vi "nanos.get.vi"(8 "error in (no error)":errorcluster, 11 "endingTimestamp in":refnum<class "endingTimestamp.lvclass">) -> (0 "error out":errorcluster, 2 "nanos":i64, 3 "endingTimestamp out":refnum<class "endingTimestamp.lvclass">)   [LabVIEW 2020, in "nominal types.lvlib" / "timestampManifest.lvlib" / "endingTimestamp.lvclass"]
uses:
  endingTimestamp.lvclass
  endingTimestamp.lvclass/endingTimestamp.ctl
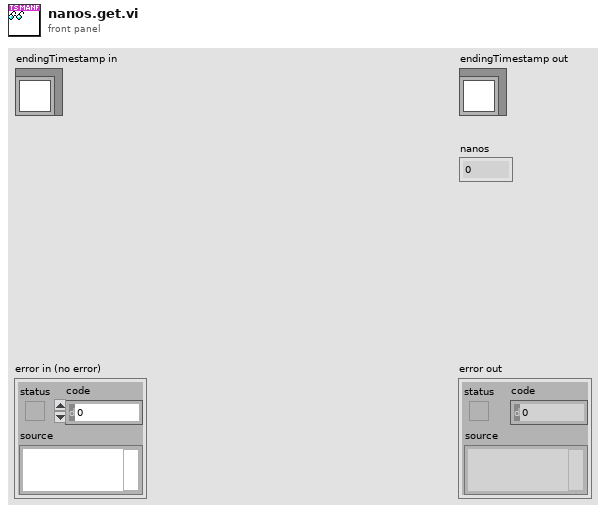
[diagram p1: front panel]
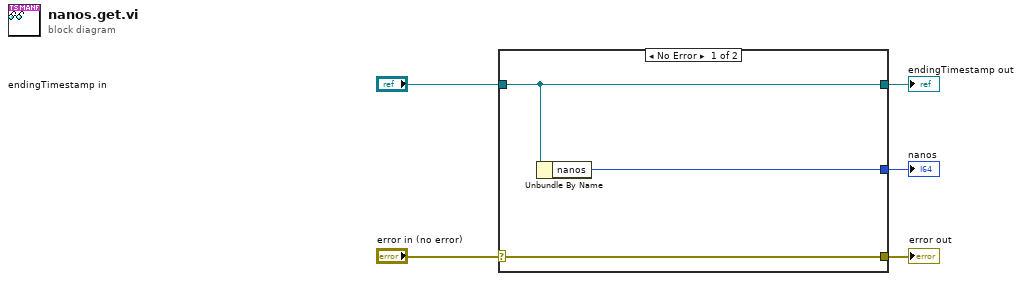
[diagram p0: block diagram]
diagram:
  n1 = case shown="No Error" "error in (no error)" {
    selector: "error in (no error)" -> [w8 w9]
    tunnel: [w8 w9] -> w4
    tunnel: [w7 w10] -> w2
    tunnel: "endingTimestamp in" -> [w7 w10]
    tunnel: [w6 _] -> w1
    frame No Error {
      n2 = Unbundle By Name(w7) -> ("nanos"=w6:i64)
    }
    frame Error {
    }
  }
  "error out" <- w4
  "endingTimestamp out" <- w2
  "nanos" <- w1
